vi "ArmExecute.vi"(8 "error in (no error)":errorcluster) -> (0 "error out":errorcluster)   [LabVIEW 2023]
doc: "Arm Execute for 2024 robot"
uses:
  ArmGetSetpointEnum.ctl
  <vilib>/Rock Robotics/WPI/ThirdParty/JAS_Junk/TrajLib/VI/BoolCmd_Recv_Internal.vi
  <vilib>/Rock Robotics/WPI/ThirdParty/JAS_Junk/TrajLib/Timer_New.vi
  <vilib>/Rock Robotics/WPI/ThirdParty/JAS_Junk/TrajLib/VI/BoolCmd_ObtainQueue.vi
  Climb/ClimbGlobal.vi
  ArmNetworkingGlobal.vi
  <vilib>/Utility/semaphor.llb/Obtain Semaphore Reference.vi
  <vilib>/Rock Robotics/WPI/ThirdParty/JAS_Junk/TrajLib/Timer_Reset.vi
  <vilib>/Rock Robotics/WPI/ThirdParty/JAS_Junk/TrajLib/Timer_Start.vi
  <vilib>/Rock Robotics/WPI/ThirdParty/JAS_Junk/TrajLib/Timer_HasPeriodPassedOnce.vi
  <vilib>/Rock Robotics/WPI/ThirdParty/JAS_Junk/TrajLib/Timer_Stop.vi
  ArmGlobal.vi
  <vilib>/Rock Robotics/WPI/ThirdParty/JAS_Junk/TrajLib/Trajectory_Library.lvlib
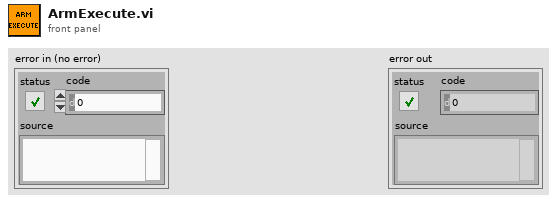
[diagram p1: front panel]
types:
  T1 = typedef "WPI_MotorControlDeviceRef.ctl" = cluster{"DeviceStatus":errorcluster, "Type":T2, "PWM":cluster{"PWM Channel":T3, "DeadBand":T4}, "CAN":cluster{"Device Number":u8, "SetOutput VI Ref":variant, "GetOutput VI Ref":variant, "Enable VI Ref":variant, "Disable VI Ref":variant, "Data":variant}, "Invert":bool, "DIO PWM":cluster{"PWM \"Enable\" Channel":T3, "DIOChannel":T5, "PWM Rate":dbl}}
  T2 = typedef "WPI_MotorControlType.ctl" = enum16{"PWM", "CAN", "DIO PWM"}
  T3 = typedef "FPGA_DIOPWMChannel.ctl" = enum8{"PWM 0", "PWM 1", "PWM 2", "PWM 3", "PWM 4", "PWM 5", "PWM 6", "PWM 7", "PWM 8", "PWM 9", "PWM MXP 0", "PWM MXP 1", "PWM MXP 2", "PWM MXP 3", "PWM MXP 4", "PWM MXP 5", "PWM MXP 6", "PWM MXP 7", "PWM MXP 8", "PWM MXP 9", "Invalid"}
  T4 = typedef "WPI_PWMDeadband.ctl" = cluster{"Name":string, "maxPositivePwm":i32, "minPositivePwm":i32, "centerPwm":i32, "maxNegativePwm":i32, "minNegativePwm":i32, "angularRange":u16}
  T5 = typedef "FPGA_DIOChannel.ctl" = enum8{"DIO 0", "DIO 1", "DIO 2", "DIO 3", "DIO 4", "DIO 5", "DIO 6", "DIO 7", "DIO 8", "DIO 9", "DIO MXP 0", "DIO MXP 1", "DIO MXP 2", "DIO MXP 3", "DIO MXP 4", "DIO MXP 5", "DIO MXP 6", "DIO MXP 7", "DIO MXP 8", "DIO MXP 9", "DIO MXP 10", "DIO MXP 11", "DIO MXP 12", "DIO MXP 13", "DIO MXP 14", "DIO MXP 15", "SPI Port CS1", "SPI Port CS2", "SPI Port CS3", "SPI Port MISO", "SPI Port MOSI", "Invalid"}
  T6 = typedef "WPI_SwitchDevRef.ctl" = cluster{"DevStatus":errorcluster, "DIO Channel":T5, "CntIndex":T7, "Normally Closed":bool}
  T7 = typedef "FPGA_CounterCtrSystemIndex.ctl" = enum8{"Ctr 0", "Ctr 1", "Ctr 2", "Ctr 3", "Ctr 4", "Ctr 5", "Ctr 6", "Ctr 7", "Invalid"}
  T8 = typedef "ArmGetSetpointEnum.ctl" = enum16{"ArmFloorPickup", "ArmAmpDeposit", "ArmSpeakerShoot", "ArmStartPosition", "ArmRestPosition", "ArmSourceIntake", "ArmAwayShoot"}
  T9 = typedef "Trajectory_Library.lvlib/PosCtrl_Tuning_Type.ctl" = cluster{"Slope":dbl, "Offset":dbl, "Error Deadband":dbl, "At Reference Count":i32, "Negate Output":bool, "Max Allowd Position":dbl, "Min Allowd Position":dbl}
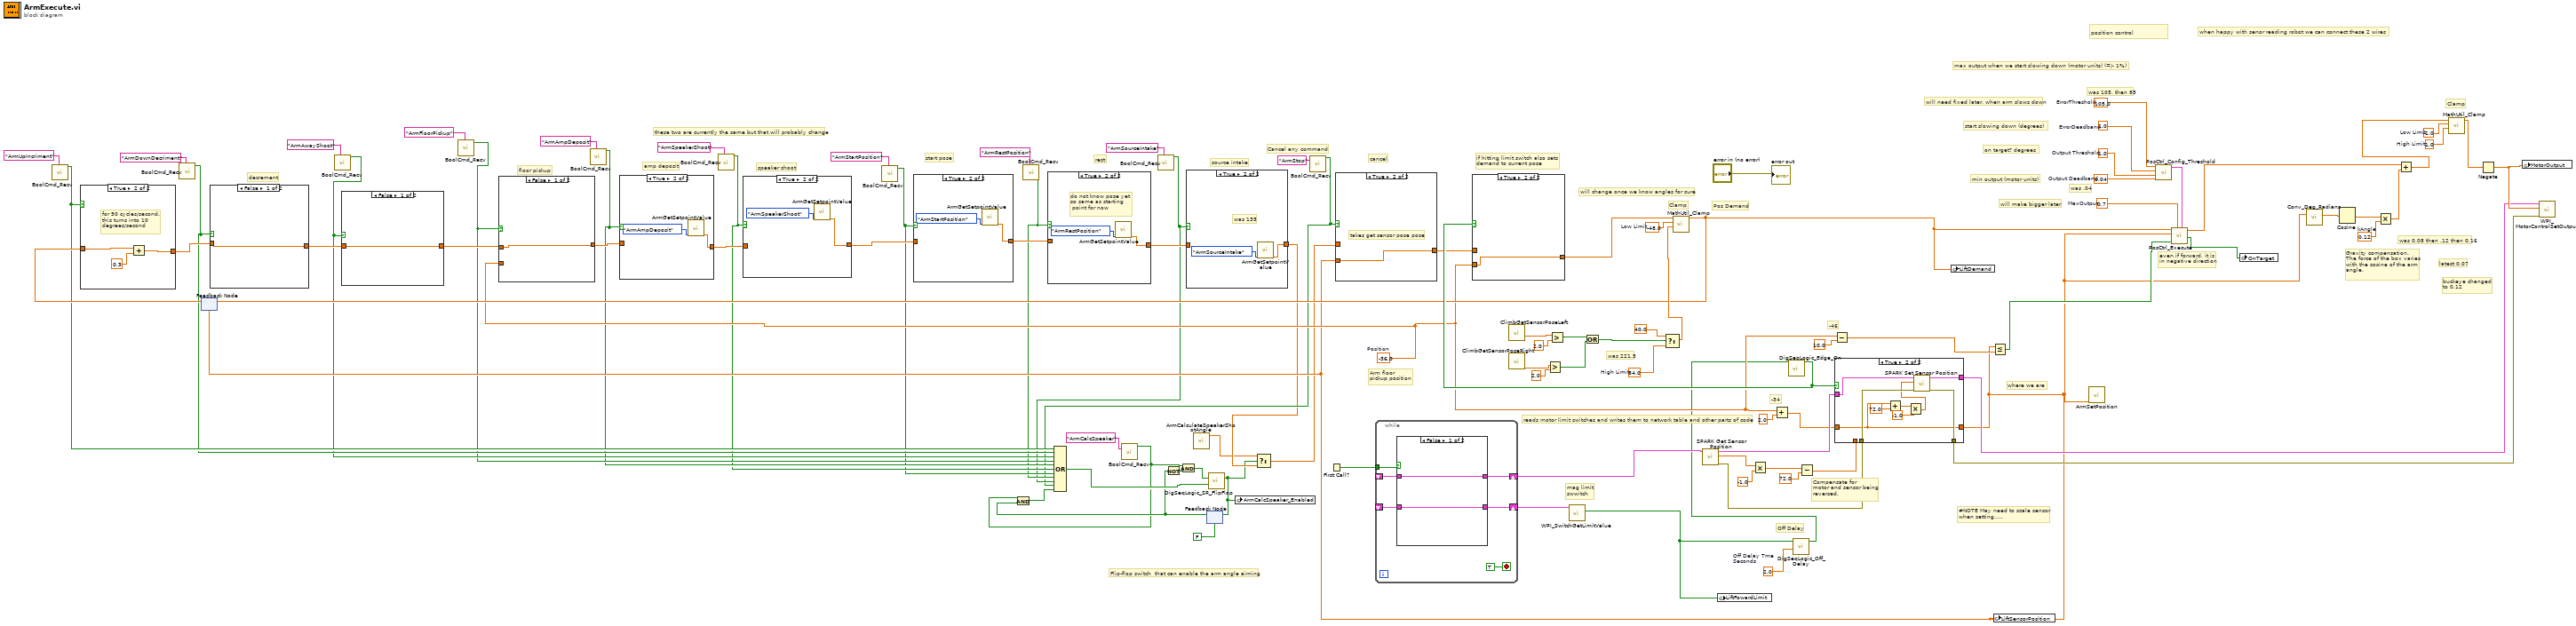
[diagram p0: block diagram]
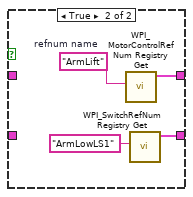
[diagram p2: hidden frame]
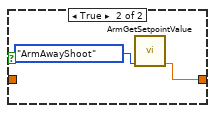
[diagram p3: hidden frame]
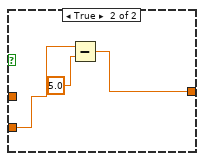
[diagram p11: hidden frame]
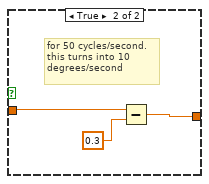
[diagram p12: hidden frame]
diagram:
  w26 = 2.0  # Off Delay Tme Seconds
  w37 = 1.0  # High Limit
  w36 = -1.0  # Low Limit
  w48 = 84.0  # High Limit
  w29 = -36.0  # Position
  w70 = 0.12  # kAngle
  w87 = -48.0  # Low Limit
  w96 = 0.7  # MaxOutput
  w94 = 105.0  # ErrorThreshold
  w93 = 1.0  # ErrorDeadband
  w92 = 1.0  # Output Threshold
  w91 = 0.04  # Output Deadband
  # "was 221.5"
  # "buckeye changed\nto 0.12"
  # "latest 0.07"
  # "Flip-flop switch  that can enable the arm angle aiming"
  # "#NOTE May need to scale sensor \nwhen setting....."
  # "Off Delay"
  # "mag limit\nswwitch"
  # "-34"
  # "-46"
  # "Pos Demand"
  # "Clamp"
  # "was 105, then 85"
  # "was .04"
  # "was 0.08 then .12 then 0.16"
  # "Arm floor\npickup position"
  # "Gravity compensation.\nThe force of the box varies\nwith the cosine of the arm\nangle."
  # "Compensate for\nmotor and sensor being\nreversed."
  # "even if forward, it is \nin negative direction"
  # "if hitting limit switch also sets \ndemand to current pose"
  # "these two are currently the same but that will probably change"
  # "Cancel any command"
  # "source intake"
  # "will change once we know angles for sure"
  # "cancel"
  # "rest"
  # "start pose"
  # "speaker shoot"
  # "Clamp"
  # "amp deposit"
  # "floor pickup"
  # "decrement"
  # "when happy with senor reading robot we can connect these 2 wires"
  # "min output (motor units)"
  # "max output when we start slowing down (motor units) (=/- 1%)"
  # "on target? degrees"
  # "start slowing down (degrees)"
  # "will make bigger later"
  # "where we are"
  # "position control"
  # "will need fixed later, when arm slows down"
  # "reads motor limit switches and writes them to network table and other parts of code"
  n1 = call <vilib>:"BoolCmd_Recv.vi"("Command Name"="ArmUpIncriment") -> ("New Request"=w19:bool)  [unwired: 9 in, 1 out]
  n2 = call <vilib>:"BoolCmd_Recv.vi"("Command Name"="ArmDownDecriment") -> ("New Request"=w18:bool)  [unwired: 9 in, 1 out]
  n3 = call <vilib>:"BoolCmd_Recv.vi"("Command Name"="ArmAwayShoot") -> ("New Request"=w17:bool)  [unwired: 9 in, 1 out]
  n4 = call <vilib>:"BoolCmd_Recv.vi"("Command Name"="ArmFloorPickup") -> ("New Request"=w16:bool)  [unwired: 9 in, 1 out]
  n5 = call <vilib>:"BoolCmd_Recv.vi"("Command Name"="ArmAmpDeposit") -> ("New Request"=w15:bool)  [unwired: 9 in, 1 out]
  n6 = call <vilib>:"BoolCmd_Recv.vi"("Command Name"="ArmSpeakerShoot") -> ("New Request"=w14:bool)  [unwired: 9 in, 1 out]
  n7 = call <vilib>:"BoolCmd_Recv.vi"("Command Name"="ArmStartPosition") -> ("New Request"=w13:bool)  [unwired: 9 in, 1 out]
  n8 = call <vilib>:"BoolCmd_Recv.vi"("Command Name"="ArmRestPosition") -> ("New Request"=w12:bool)  [unwired: 9 in, 1 out]
  n9 = call <vilib>:"BoolCmd_Recv.vi"("Command Name"="ArmCalcSpeaker") -> ("New Request"=w4:bool)  [unwired: 9 in, 1 out]
  n10 = call <vilib>:"BoolCmd_Recv.vi"("Command Name"="ArmSourceIntake") -> ("New Request"=w11:bool)  [unwired: 9 in, 1 out]
  n11 = call "ArmCalculateSpeakerShootAngle.vi"() -> ("ArmAngle (degrees)"=w7:dbl)  [unwired: 11 in]
  n12 = feedback #1(FALSE ("Output")) -> (w5:bool)
  n13 = And(x=w4, y=w5) -> (x .and. y?=w3:bool)
  n14 = Not(x=w5) -> (.not. x?=w21:bool)
  n15 = And(x=w4, y=w21) -> (x .and. y?=w20:bool)
  n16 = call <vilib>:"BoolCmd_Recv.vi"("Command Name"="ArmStop") -> ("New Request"=w10:bool)  [unwired: 9 in, 1 out]
  n17 = Compound Arithmetic op=OR(w19, w18, w17, w16, w15, w14, w13, w12, w11, w10, w3) -> (w6:bool)
  n18 = call <vilib>:"DigSeqLogic_SR_FlipFlop.vi"("Set"=w20, "Reset"=w6) -> ("Output"=w1:bool)  [unwired: 12 in, 1 out]
  n19 = feedback-in #1(w1) -> ()
  n20 = global write "ArmGlobal.vi" "ArmCalcSpeaker_Enabled"(w1) -> ()
  n21 = First Call?() -> (First Call?: T/F=w45:bool)
  n22 = while {
    tunnel: w45 -> [w101]
    shift-right: [w102] -> w38
    shift-left: _ -> [w99]
    shift-right: [w98] -> w41
    shift-left: _ -> [w97]
    stop <- TRUE stop-if-true
    n23 = case shown="False" w101 {
      tunnel: [w104 w108] -> w102
      tunnel: w99 -> [w104 _]
      tunnel: [w103 w105] -> w98
      tunnel: w97 -> [w103 _]
      frame False {
      }
      frame True {
        w107 = "ArmLift"  # refnum name
        n24 = call <vilib>:"WPI_MotorControlRefNum Registry Get.vi"("refnum name"=w107) -> ("MotorControlDevRef"=w108:T1)  [unwired: 9 in, 1 out]
        n25 = call <vilib>:"WPI_SwitchRefNum Registry Get.vi"("refnum name"="ArmLowLS1") -> ("SwitchDevRef"=w105:T6)  [unwired: 9 in, 1 out]
      }
    }
  }
  n26 = call "ClimbGetSensorPoseRight.vi"() -> ("ClimbGetSensorPoseRight"=w52:dbl)  [unwired: 11 in]
  n27 = call "ClimbGetSensorPoseLeft.vi"() -> ("ClimbGetSensorPoseLeft"=w55:dbl)  [unwired: 11 in]
  n28 = Greater?(x=w52, y=2.0) -> (0:w50:bool)
  n29 = Greater?(x=w55, y=2.0) -> (0:w51:bool)
  n30 = call <vilib>:"WPI_SwitchGetLimitValue.vi"("SwitchDevRef"=w41) -> ("Switch Pressed"=w25:bool)  [unwired: 8 in, 2 out]
  n31 = Or(x=w51, y=w50) -> (x .or. y?=w49:bool)
  n32 = Select(t=40.0, s=w49, f=w48) -> (s? t:f=w46:dbl)
  n33 = call <vilib>:"SPARK Get Sensor Position.vi"("MotorControlDevRef in"=w38) -> ("error out"=w44:errorcluster, "Sensor Position"=w66:dbl, "MotorControlDevRef out"=w67:T1)  [unwired: 7 in, 1 out]
  n34 = global write "ArmNetworkingGlobal.vi" "LiftFowardLimit"(w25) -> ()
  n35 = Multiply(x=w66, y=-1.0) -> (x*y=w64:dbl)
  n36 = Add(x=w29, y=2.0) -> (x+y=w32:dbl)
  n37 = call <vilib>:"DigSeqLogic_Off_Delay.vi"("Delay"=w26, "Input"=w25) -> ("Output"=w24:bool)  [unwired: 8 in, 1 out]
  n38 = call <vilib>:"DigSeqLogic_Edge_On.vi"("Input"=w24) -> ("On Edge"=w61:bool)  [unwired: 10 in]
  n39 = Subtract(x=w64, y=72.0) -> (x-y=w62:dbl)
  n40 = Subtract(x=w29, y=10.0) -> (x-y=w27:dbl)
  n41 = case shown="True" w61 {
    tunnel: [w110 w120] -> w40
    tunnel: [w111 w116] -> w23
    tunnel: w62 -> [w111 _]
    tunnel: w67 -> [w110 w119]
    tunnel: w32 -> [_ w116]
    tunnel: w44 -> [w109 w118]
    tunnel: [w109 w117] -> w39
    frame False {
    }
    frame True {
      n42 = Add(x=w116, y=72.0) -> (x+y=w115:dbl)
      n43 = Multiply(x=w115, y=-1.0) -> (x*y=w112:dbl)
      n44 = call <vilib>:"SPARK Set Sensor Position.vi"("error in"=w118, "Position"=w112, "MotorControlDeviceRef"=w119) -> ("error out"=w117:errorcluster, "MotorControlDeviceRef"=w120:T1)  [unwired: 7 in]
    }
  }
  n45 = feedback #2(w23) -> (w90:dbl)
  n46 = case shown="True" w19 {
    tunnel: w90 -> [w121 w124]
    tunnel: [w121 w122] -> w89
    frame False {
    }
    frame True {
      # "for 50 cycles/second.\nthis turns into 10 \ndegrees/second"
      n47 = Add(x=w124, y=0.3) -> (x+y=w122:dbl)
    }
  }
  n48 = case shown="False" w18 {
    tunnel: w89 -> [w125 w127]
    tunnel: [w125 w126] -> w58
    frame False {
    }
    frame True {
      # "for 50 cycles/second.\nthis turns into 10 \ndegrees/second"
      n49 = Subtract(x=w127, y=0.3) -> (x-y=w126:dbl)
    }
  }
  n50 = case shown="False" w17 {
    tunnel: w58 -> [w129 _]
    tunnel: [w129 w130] -> w57
    frame False {
    }
    frame True {
      n51 = call "ArmGetSetpointValue.vi"("ArmSetpoints"=ArmGetSetpointEnum."ArmAwayShoot") -> ("Setpoint"=w130:dbl)  [unwired: 10 in]
    }
  }
  n52 = case shown="False" w16 {
    tunnel: w57 -> [w132 _]
    tunnel: [w132 w134] -> w88
    tunnel: w29 -> [_ w135]
    frame False {
    }
    frame True {
      n53 = Subtract(x=w135, y=5.0) -> (x-y=w134:dbl)
    }
  }
  n54 = case shown="True" w15 {
    tunnel: w88 -> [w136 _]
    tunnel: [w136 w137] -> w86
    frame False {
    }
    frame True {
      n55 = call "ArmGetSetpointValue.vi"("ArmSetpoints"=ArmGetSetpointEnum."ArmAmpDeposit") -> ("Setpoint"=w137:dbl)  [unwired: 10 in]
    }
  }
  n56 = case shown="True" w14 {
    tunnel: w86 -> [w139 _]
    tunnel: [w139 w140] -> w85
    frame False {
    }
    frame True {
      n57 = call "ArmGetSetpointValue.vi"("ArmSetpoints"=ArmGetSetpointEnum."ArmSpeakerShoot") -> ("Setpoint"=w140:dbl)  [unwired: 10 in]
    }
  }
  n58 = case shown="True" w13 {
    tunnel: w85 -> [w142 _]
    tunnel: [w142 w143] -> w84
    frame False {
    }
    frame True {
      n59 = call "ArmGetSetpointValue.vi"("ArmSetpoints"=ArmGetSetpointEnum."ArmStartPosition") -> ("Setpoint"=w143:dbl)  [unwired: 10 in]
    }
  }
  n60 = case shown="True" w12 {
    tunnel: w84 -> [w145 _]
    tunnel: [w145 w146] -> w83
    frame False {
    }
    frame True {
      # "do not know pose yet \nso same as starting\n point for now"
      n61 = call "ArmGetSetpointValue.vi"("ArmSetpoints"=ArmGetSetpointEnum."ArmRestPosition") -> ("Setpoint"=w146:dbl)  [unwired: 10 in]
    }
  }
  n62 = case shown="True" w11 {
    tunnel: w83 -> [w148 _]
    tunnel: [w148 w149] -> w9
    frame False {
    }
    frame True {
      # "was 135"
      n63 = call "ArmGetSetpointValue.vi"("ArmSetpoints"=ArmGetSetpointEnum."ArmSourceIntake") -> ("Setpoint"=w149:dbl)  [unwired: 10 in]
    }
  }
  n64 = Select(t=w7, s=w1, f=w9) -> (s? t:f=w8:dbl)
  n65 = case shown="True" w10 {
    tunnel: w8 -> [w151 _]
    tunnel: [w151 w152] -> w59
    tunnel: w23 -> [_ w152]
    frame False {
    }
    frame True {
      # "takes get sensor pose pose"
    }
  }
  n66 = case shown="True" w61 {
    tunnel: w29 -> [_ w154]
    tunnel: [w153 w154] -> w60
    tunnel: w59 -> [w153 _]
    frame False {
    }
    frame True {
    }
  }
  n67 = call <vilib>:"MathUtil_Clamp.vi"("High Limit"=w46, "Low Limit"=w87, "Value"=w60) -> ("Result"=w33:dbl)  [unwired: 8 in]
  n68 = feedback-in #2(w33) -> ()
  n69 = global write "ArmNetworkingGlobal.vi" "LiftDemand"(w33) -> ()
  n70 = Less Or Equal?(x=w23, y=w27) -> (x <= y?=w30:bool)
  n71 = global write "ArmNetworkingGlobal.vi" "LiftSensorPosition"(w23) -> ()
  n72 = call "ArmSetPosition.vi"("ArmPos"=w23) -> ()  [unwired: 11 in]
  n73 = call <vilib>:"PosCtrl_Config_Threshold.vi"("Output Deadband"=w91, "Output Threshold"=w92, "ErrorDeadband"=w93, "ErrorThreshold"=w94) -> ("PosCtrl_Config_Params"=w95:T9)  [unwired: 7 in]
  n74 = call <vilib>:"PosCtrl_Execute.vi"("PosCtrl_Config_Params"=w95, "MaxOutput"=w96, "Rev Limit Switch"=w30, "CurrentPosition"=w23, "TargetPosition"=w33) -> ("OnTarget"=w42:bool, "Output"=w72:dbl)  [unwired: 4 in, 1 out]
  n75 = global write "ArmNetworkingGlobal.vi" "OnTarget"(w42) -> ()
  n76 = call <vilib>:"Conv_Deg_Radians.vi"("Degress"=w23) -> ("Radians"=w68:dbl)  [unwired: 10 in]
  n77 = Cosine(x=w68) -> (cos(x)=w69:dbl)
  n78 = Multiply(x=w69, y=w70) -> (x*y=w71:dbl)
  n79 = Add(x=w72, y=w71) -> (x+y=w35:dbl)
  n80 = call <vilib>:"MathUtil_Clamp.vi"("High Limit"=w37, "Low Limit"=w36, "Value"=w35) -> ("Result"=w34:dbl)  [unwired: 8 in]
  n81 = Negate(x=w34) -> (-x=w43:dbl)
  n82 = global write "ArmNetworkingGlobal.vi" "MotorOutput"(w43) -> ()
  n83 = call <vilib>:"WPI_MotorControlSetOutput.vi"("error in (no error)"=w39, "Output"=w43, "MotorControlDevRef"=w40) -> ()  [unwired: 6 in, 3 out]
  "error out" <- "error in (no error)"
